vi "GetChannelByIndex.vi"(8 "error in (no error)":errorcluster, 9 "index of element":i32, 11 "ChanGrp in":refnum<class "ChanGrp.lvclass">) -> (0 "error out":errorcluster, 3 "Channel":refnum<class "Channel.lvclass">)   [LabVIEW 2012, in "Configuration Grandmaster.lvlib" / "ChanGrp.lvclass"]
uses:
  ChanGrp.lvclass
  Measurements/Class Channel/Channel.lvclass
  ChanGrp.lvclass/ChanGrp.ctl
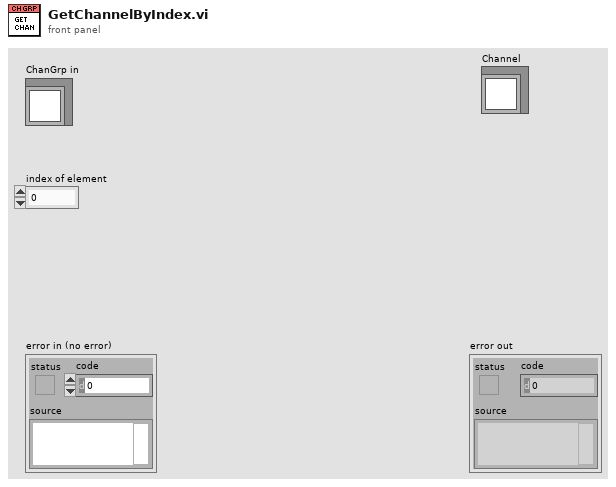
[diagram p1: front panel]
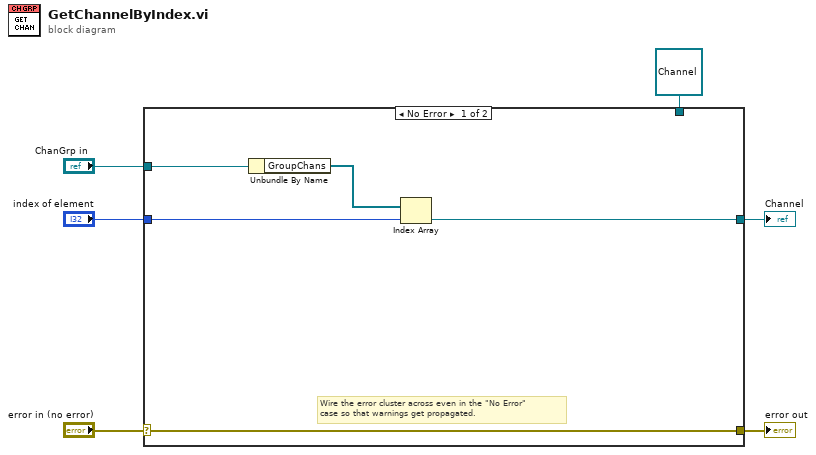
[diagram p0: block diagram]
diagram:
  n1 = case shown="No Error" "error in (no error)" {
    selector: "error in (no error)" -> [w11 w13]
    tunnel: [w11 w13] -> w5
    tunnel: "ChanGrp in" -> [w10 _]
    tunnel: "index of element" -> [w8 _]
    tunnel: [w7 w12] -> w2
    tunnel: refnum<class "Channel.lvclass"> refnum ("Measurement.lvclass") -> [_ w12]
    frame No Error {
      # "Wire the error cluster across even in the \"No Error\"\ncase so that warnings get propagated."
      n2 = Unbundle By Name(w10) -> ("GroupChans"=w9:refnum<class "Channel.lvclass">[])
      n3 = Index Array(array=w9, index=w8) -> (element=w7:refnum<class "Channel.lvclass">)
    }
    frame Error {
    }
  }
  "error out" <- w5
  "Channel" <- w2
